vi "Object tracking.vi"(7 "Tracking Ops":T5(ring), 8 "error in (no error)":errorcluster, 9 "Rectangle":T7={"Left"=183, "Top"=90, "Right"=199, "Bottom"=108, "Rotation"=0.0} {"Rotation" format="%.2f"; "Left" scale=0.0..1024.0; "Right" scale=0.0..1024.0}, 10 "Shape Adapted Options in":T4={"Number of Histogram Bins"=8, "Blending Parameter (%)"=10.0, "Max Scale Change (%)"=1.0, "Max Rotation Change"=40.0, "Max Shape Change (%)"=1.0, "Maximum Iterations"=15}, 11 "Image IN":T2(plugin-control)) -> (0 "error out":errorcluster, 1 "Objects found":T3(array[cluster]), 2 "Object Tracking Session Out":T6, 3 "Image OUT":T2(plugin-control), 4 "Bounding Box":cluster{"X":dbl, "Y":dbl}[](array[cluster]), 5 "Object Found?":bool, 6 "Location":cluster{"X":dbl, "Y":dbl})   [LabVIEW 2020]
uses:
  <vilib>/vision/Tracking.llb/IMAQ Object Tracking Session.ctl
  <vilib>/vision/Image Controls.llb/IMAQ Image.ctl
panel:
  in  "Mean Shift Options in":T1={"Number of Histogram Bins"=8, "Blending Parameter (%)"=10.0, "Maximum Iterations"=15}
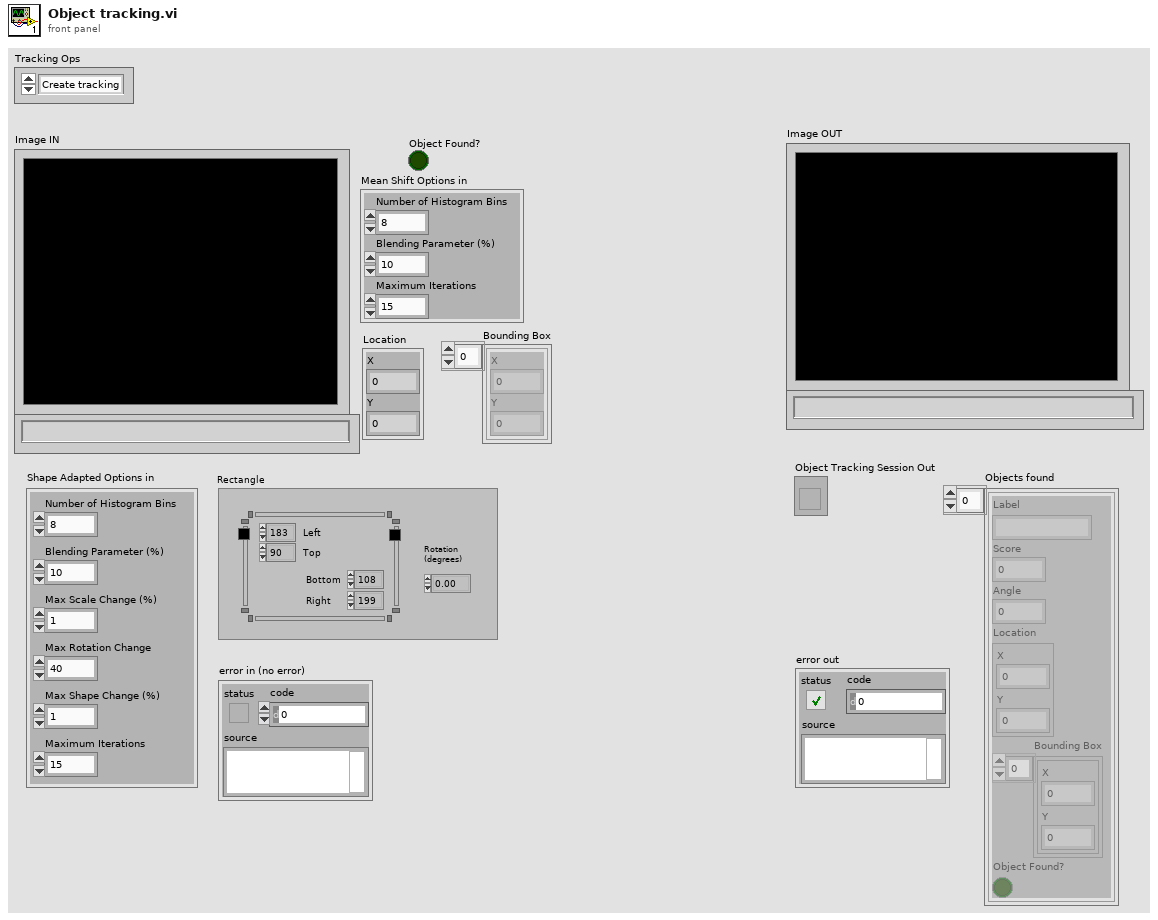
[diagram p1: front panel]
types:
  T1 = cluster{"Number of Histogram Bins":i32, "Blending Parameter (%)":dbl, "Maximum Iterations":i32}
  T2 = typedef "IMAQ Image.ctl" = refnum<image>
  T3 = cluster{"Label":string, "Score":i32, "Angle":dbl, "Location":cluster{"X":dbl, "Y":dbl}, "Bounding Box":cluster{"X":dbl, "Y":dbl}[], "Object Found?":bool}[]
  T4 = cluster{"Number of Histogram Bins":i32, "Blending Parameter (%)":dbl, "Max Scale Change (%)":dbl, "Max Rotation Change":dbl, "Max Shape Change (%)":dbl, "Maximum Iterations":i32}
  T5 = enum16{"Create tracking", "Setup Object", "Track Object", "Close"}
  T6 = typedef "IMAQ Object Tracking Session.ctl" = refnum<k20>
  T7 = typedef "IMAQ Rectangle" = cluster{"Left":i32, "Top":i32, "Right":i32, "Bottom":i32, "Rotation":dbl}
  T8 = typedef "ROI Descriptor" = cluster{"Global Rectangle":i32[], "Contours":cluster{"ID":enum32{"External", "Internal"}, "Type":u32, "Coordinates":i32[]}[]}
  T9 = cluster{"Label":string, "Score":i32, "Angle":dbl, "Location":cluster{"X":dbl, "Y":dbl}, "Bounding Box":cluster{"X":dbl, "Y":dbl}[], "Object Found?":bool}
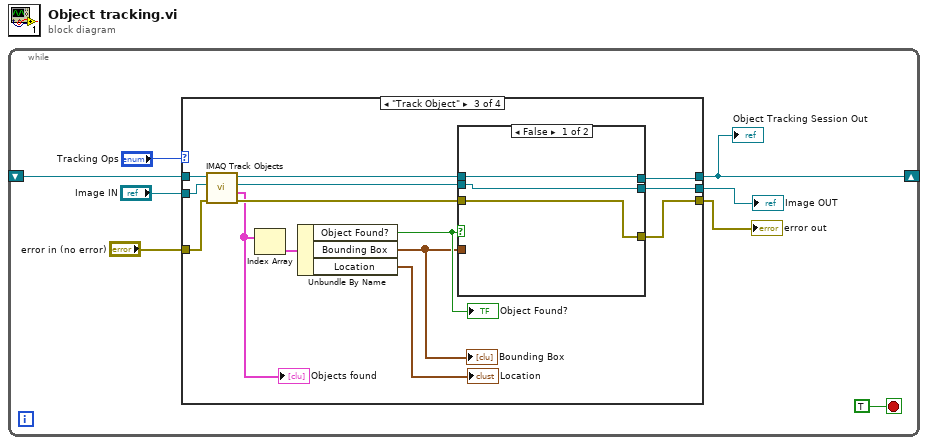
[diagram p0: block diagram]
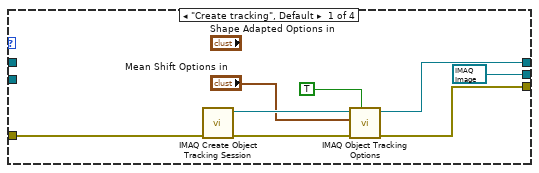
[diagram p2: hidden frame]
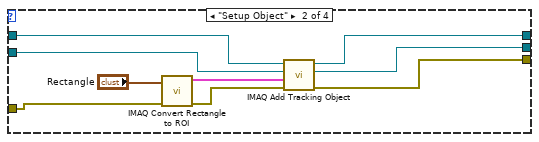
[diagram p3: hidden frame]
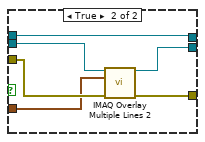
[diagram p4: hidden frame]
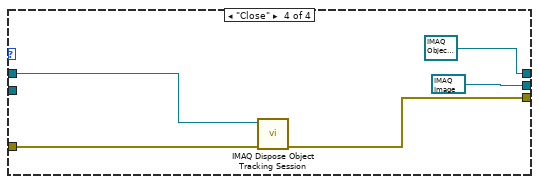
[diagram p5: hidden frame]
diagram:
  n1 = while {
    shift-right: [w5] -> _
    shift-left: _ -> [w4]
    stop <- TRUE stop-if-true
    n2 = case shown="\"Track Object\"" "Tracking Ops" {
      tunnel: [w11 w23 w29 T6 refnum ("Object Tracking Session Out")] -> w5
      tunnel: [w12 w22 w28 w51] -> w8
      tunnel: "error in (no error)" -> [w13 w18 w38 w53]
      tunnel: w4 -> [_ w21 w39 w52]
      tunnel: "Image IN" -> [_ w19 w37 _]
      tunnel: [T2 refnum ("Image Out") w17 w30 T2 refnum ("Image Out")] -> w1
      frame "Create tracking", Default {
        n3 = call "IMAQ Create Object Tracking Session"("error in (no error)"=w13) -> ("error out"=w14:errorcluster, "Object Tracking Session"=w16:T6)  [unwired: 9 out]
        n4 = call-poly "IMAQ Object Tracking Options"("Get/Set (Get)"=TRUE, "error in (no error)"=w14, "Mean Shift Options in"="Mean Shift Options in", "Object Tracking Session In"=w16) -> ("error out"=w12:errorcluster, "Object Tracking Session Out"=w11:T6)  [unwired: 5 in, 1 out]
      }
      frame "Setup Object" {
        n5 = call "IMAQ Convert Rectangle to ROI"("error in (no error)"=w18, "Rectangle"="Rectangle") -> ("error out"=w24:errorcluster, "ROI Descriptor"=w25:T8)  [unwired: 7 in]
        n6 = call "IMAQ Add Tracking Object"("error in (no error)"=w24, "ROI Descriptor"=w25, "Image"=w19, "Object Tracking Session In"=w21) -> ("error out"=w22:errorcluster, "Image (duplicate)"=w17:T2, "Object Tracking Session Out"=w23:T6)  [unwired: 1 in, 4 out]
      }
      frame "Track Object" {
        n7 = call "IMAQ Track Objects"("error in (no error)"=w38, "Image"=w37, "Object Tracking Session In"=w39) -> ("error out"=w33:errorcluster, "Objects (pixel)"=w27:T3, "Image (duplicate)"=w34:T2, "Object Tracking Session Out"=w32:T6)  [unwired: 1 in, 4 out]
        "Objects found" <- w27
        n8 = Index Array(array=w27) -> (element=w36:T9)  [unwired: 1 in]
        n9 = Unbundle By Name(w36) -> ("Object Found?"=w35:bool, "Bounding Box"=w31:cluster{"X":dbl, "Y":dbl}[], "Location"=→"Location":cluster{"X":dbl, "Y":dbl})
        "Object Found?" <- w35
        "Bounding Box" <- w31
        n10 = case shown="False" w35 {
          tunnel: w34 -> [w41 w47]
          tunnel: w33 -> [w40 w48]
          tunnel: w32 -> [w42 w44]
          tunnel: w31 -> [_ w46]
          tunnel: [w41 w45] -> w30
          tunnel: [w42 w44] -> w29
          tunnel: [w40 w43] -> w28
          frame False {
          }
          frame True {
            n11 = call "IMAQ Overlay Multiple Lines 2"("Image"=w47, "Line End Points"=w46, "error in (no error)"=w48) -> ("Image Out"=w45:T2, "error out"=w43:errorcluster)  [unwired: 5 in, 6 out]
          }
        }
      }
      frame "Close" {
        n12 = call "IMAQ Dispose Object Tracking Session"("error in (no error)"=w53, "Object Tracking Session"=w52) -> ("error out"=w51:errorcluster)  [unwired: 9 out]
      }
    }
    "Object Tracking Session Out" <- w5
    "error out" <- w8
    "Image OUT" <- w1
  }
